vi "Scrape Matplotlib Color Map Hacking (single).vi"() -> ()   [LabVIEW 2019]
uses:
  <vilib>/Utility/sysdir.llb/System Directory Type.ctl
panel:
  out "Array":u32[](array[colorbox])
  out "Intensity Graph 2":dbl[][](graph)
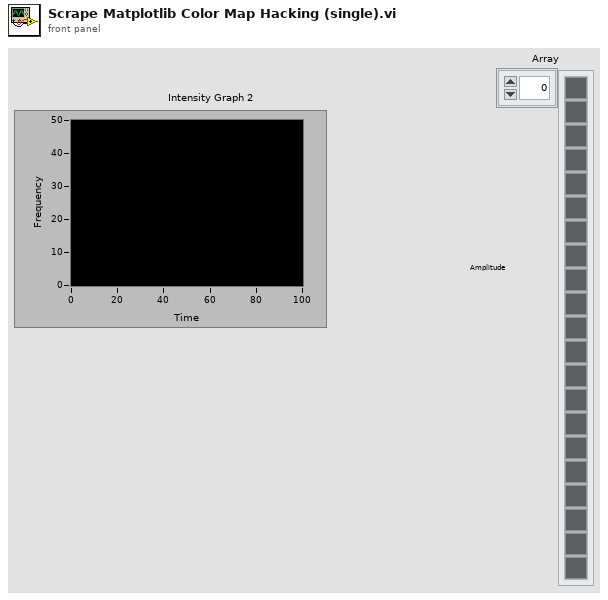
[diagram p1: front panel]
types:
  T1 = enum16{"open", "replace", "create", "open or create", "replace or create", "replace or create with confirmation"}
  T2 = typedef "System Directory Type.ctl" = i32
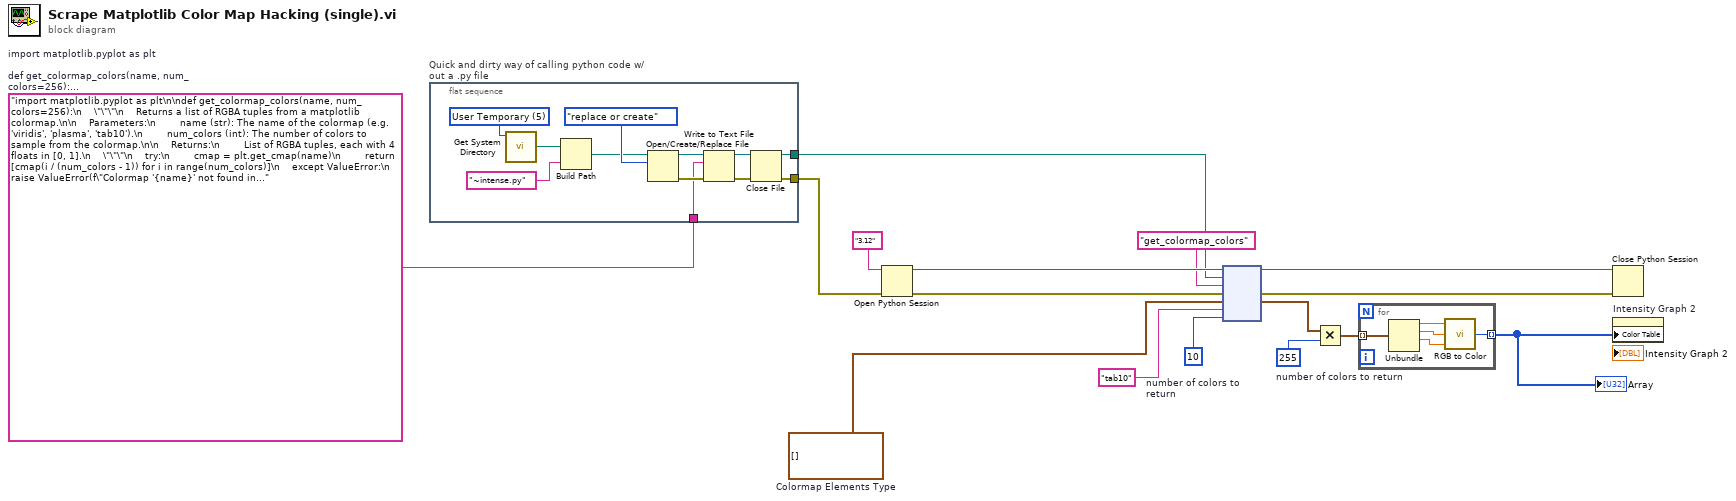
[diagram p0: block diagram]
diagram:
  w1 = 255  # number of colors to return
  w4 = 10  # number of colors to return
  w8 = cluster{"R":dbl, "G":dbl, "B":dbl, "A":dbl}[] []  # Colormap Elements Type
  w9 = "import matplotlib.pyplot as plt\n\ndef get_colormap_colors(name, num_colors=256):\n    \"\"\"\n    Returns a list of RGBA tuples from a matplotlib colormap.\n\n    Parameters:\n        name (str): The name of the colormap (e.g. 'viridis', 'plasma', 'tab10').\n        num_colors (int): The number of colors to sample from the colormap.\n\n    Returns:\n        List of RGBA tuples, each with 4 floats in [0, 1].\n    \"\"\"\n    try:\n        cmap = plt.get_cmap(name)\n        return [cmap(i / (num_colors - 1)) for i in range(num_colors)]\n    except ValueError:\n        raise ValueError(f\"Colormap '{name}' not found in matplotlib.\")\n\ndef get_colormaps():\n    colormaps = plt.colormaps()\n    return colormaps\n"  # import matplotlib.pyplot as plt  def get_colormap_colors(name, num_colors=256):     """     Returns a list of RGBA tuples from a matplotlib colormap.      Parameters:         name (str): The name of the colormap (e.g. 'viridis', 'plasma', 'tab10').         num_colors (int): The number of colors to sample from the colormap.      Returns:         List of RGBA tuples, each with 4 floats in [0, 1].     """     try:         cmap = plt.get_cmap(name)         return [cmap(i / (num_colors - 1)) for i in range(num_colors)]     except ValueError:         raise ValueError(f"Colormap '{name}' not found in matplotlib.")  def get_colormaps():     colormaps = plt.colormaps()     return colormaps
  n1 = flat-sequence "Quick and dirty way of calling python code w/out a .py file" {
    tunnel: [w26] -> w15
    tunnel: [w20] -> w13
    tunnel: w9 -> [w17]
    frame #0 {
      w19 = T2 5 items=["User Home"=0, "User Desktop"=1, "User Documents"=2, "User Application Data"=3, "User Preferences"=4, "User Temporary"=5, "Public Documents"=6, "Public Application Data"=7, "Public Preferences"=8, "Public Cache"=13, "System Core Libraries"=9, "System Installed Libraries"=10, "Application Files"=11, "Boot Volume Root"=12] ("system directory type")
      n2 = call <vilib>:"Get System Directory.vi"("system directory type"=w19) -> ("system directory"=w22:path)  [unwired: 10 in]
      n3 = Build Path(base path=w22, name or relative path="~intense.py") -> (appended path=w21:path)
      n4 = Open/Create/Replace File(file path (use dialog)=w21, operation (0:open)=T1."replace or create") -> (refnum out=w25:refnum<file>, error out=w24:errorcluster)  [unwired: 4 in, 1 out]
      n5 = Write to Text File(file (use dialog)=w25, text=w17, error in=w24) -> (refnum out=w27:refnum<file>, error out=w28:errorcluster)  [unwired: 1 in, 1 out]
      n6 = Close File(refnum=w27, error in=w28) -> (path=w20:path, error out=w26:errorcluster)
    }
  }
  n7 = Open Python Session(python version="3.12" ("Python version"), 3:w15) -> (session out=w14:refnum<k35>, error out=w16:errorcluster)  [unwired: 1 in]
  n8 = node(w14, w13, "get_colormap_colors" ("function name"), w16, w8, "tab10" ("function name"), w4) -> (w12:refnum<k35>, w11:errorcluster, w6:cluster{"R":dbl, "G":dbl, "B":dbl, "A":dbl}[])  [unwired: 2 in, 2 out]
  n9 = Multiply(x=w6, y=w1) -> (x*y=w5:cluster{"R":dbl, "G":dbl, "B":dbl, "A":dbl}[])
  n10 = for {
    tunnel: w5 -> [w33] mode=indexing
    tunnel: [w29] -> w2 mode=indexing
    n11 = Unbundle(w33) -> ("R"=w32:dbl, "G"=w31:dbl, "B"=w30:dbl)  [unwired: 1 out]
    n12 = call <vilib>:"RGB to Color.vi"("B"=w30, "G"=w31, "R"=w32) -> ("Color"=w29:u32)
  }
  "Array" <- w2
  n13 = Close Python Session(session in=w12, error in=w11) -> ()  [unwired: 1 out]
  n14 = property on="Intensity Graph 2" class="IntGraph (strict)"("Color Table"=w2) -> ()  [unwired: 2 in, 2 out]
